vi "lvgit commit.vi"(8 "error in":errorcluster, 11 "path":path) -> (0 "error out":errorcluster)   [LabVIEW 2017]
uses:
  <vilib>/Hampel Software Engineering/Git API/Git API/GIT-api.lvclass/GIT-api.ctl
  <vilib>/Hampel Software Engineering/Git API/Git API/GIT-api.lvclass
panel:
  out "Staged Files":string[](array[string])
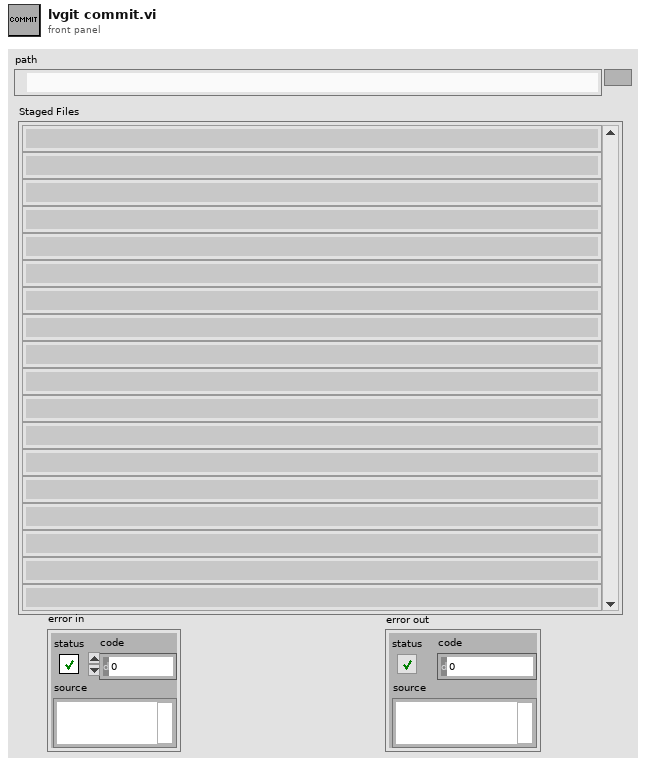
[diagram p1: front panel]
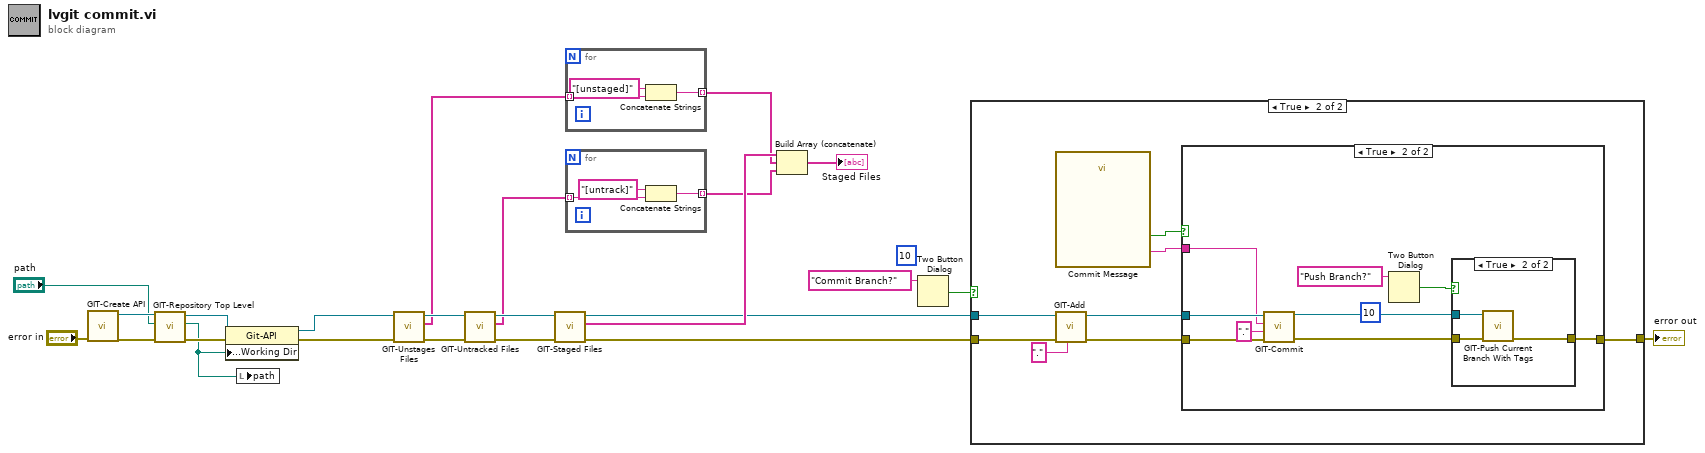
[diagram p0: block diagram]
diagram:
  (unwired) 10 ("F Timeout(-1 s)")
  n1 = call <vilib>:"GIT-Create API.vi"("error in"="error in") -> ("error out"=w21:errorcluster, "git-api out"=w22:refnum<class "GIT-api.lvclass">)  [unwired: 9 in]
  n2 = call <vilib>:"GIT-Repository Top Level.vi"("error in"=w21, "Current Path"="path", "git-api in"=w22) -> ("error out"=w24:errorcluster, "Repo Top Level Path"=w19:path, "git-api out"=w23:refnum<class "GIT-api.lvclass">)  [unwired: 6 in]
  n3 = property class="Git-API"(reference=w23, error in=w24, "Accessors:Working Dir"=w19) -> (reference out=w7:refnum<class "GIT-api.lvclass">, error out=w8:errorcluster)
  n4 = local write "path"(w19) -> ()
  n5 = call <vilib>:"GIT-Unstages Files.vi"("error in"=w8, "Git-API in"=w7) -> ("error out"=w16:errorcluster, "Unstaged Files"=w13:string[], "Git-API out"=w17:refnum<class "GIT-api.lvclass">)  [unwired: 7 in]
  n6 = call <vilib>:"GIT-Untracked Files.vi"("error in"=w16, "Git-API in"=w17) -> ("error out"=w15:errorcluster, "Untracked Files"=w12:string[], "Git-API out"=w14:refnum<class "GIT-api.lvclass">)  [unwired: 7 in]
  n7 = call <vilib>:"GIT-Staged Files.vi"("error in"=w15, "Git-API in"=w14) -> ("error out"=w6:errorcluster, "Staged Files"=w18:string[], "Git-API out"=w5:refnum<class "GIT-api.lvclass">)  [unwired: 7 in]
  n8 = for {
    tunnel: w13 -> [w27] mode=indexing
    tunnel: [w25] -> w10 mode=indexing
    n9 = Concatenate Strings("[unstaged]" ("string"), w27) -> (w25:string)
  }
  n10 = for {
    tunnel: w12 -> [w30] mode=indexing
    tunnel: [w28] -> w9 mode=indexing
    n11 = Concatenate Strings("[untrack]" ("string"), w30) -> (w28:string)
  }
  n12 = Build Array (concatenate)(w18, w10, w9) -> (→"Staged Files":string[])
  n13 = Two Button Dialog(message="Commit Branch?") -> (T button?=w3:bool)  [unwired: 2 in]
  n14 = case shown="True" w3 {
    tunnel: [w31 w37] -> w2
    tunnel: w5 -> [_ w35]
    tunnel: w6 -> [w31 w34]
    frame False {
    }
    frame True {
      n15 = call "Commit Message"() -> ("Message"=w39:string, "OK"=w38:bool)  [unwired: 17 in, 1 out]
      n16 = call <vilib>:"GIT-Add.vi"("param"=".", "error in"=w34, "git-api in"=w35) -> ("error out"=w33:errorcluster, "git-api out"=w32:refnum<class "GIT-api.lvclass">)  [unwired: 6 in, 1 out]
      n17 = case shown="True" w38 {
        tunnel: [w40 w44] -> w37
        tunnel: w32 -> [_ w49]
        tunnel: w33 -> [w40 w48]
        tunnel: w39 -> [_ w46]
        frame False {
        }
        frame True {
          (unwired) 10 ("F Timeout(-1 s)")
          n18 = call <vilib>:"GIT-Commit.vi"("error in"=w48, "params"=".", "msg"=w46, "Git-API in"=w49) -> ("error out"=w45:errorcluster, "Git-API out"=w43:refnum<class "GIT-api.lvclass">)  [unwired: 6 in]
          n19 = Two Button Dialog(message="Push Branch?") -> (T button?=w41:bool)  [unwired: 2 in]
          n20 = case shown="True" w41 {
            tunnel: w45 -> [w50 w53]
            tunnel: [w50 w52] -> w44
            tunnel: w43 -> [_ w51]
            frame False {
            }
            frame True {
              n21 = call <vilib>:"GIT-Push Current Branch With Tags.vi"("error in"=w53, "Git-API in"=w51) -> ("error out"=w52:errorcluster)  [unwired: 8 in, 1 out]
            }
          }
        }
      }
    }
  }
  "error out" <- w2
